vi "StateMachine.vi"() -> ()   [LabVIEW 2017]
uses:
  StateMachineController.ctl
  <vilib>/measure/mascope.llb/Amplitude and Levels 1 chan.vi
  <vilib>/Analysis/NI_AALBase.lvlib
  <vilib>/measure/NI_MAPro.lvlib
panel:
  in  "state settings":T1={"method"=enum."auto select", "histogram size"=256, "histogram method"=enum."mode", "reserved"=1.0} {"reserved" format="%0.2f"}
  out "high state level":dbl format="%.2g"
  out "amplitude":dbl format="%.2p"
  in  "Amplitude":dbl
  in  "stop":bool
  in  "Analyze Data":bool
  in  "Acquire Data":bool
  out "Waveform Graph":dbl[](graph)
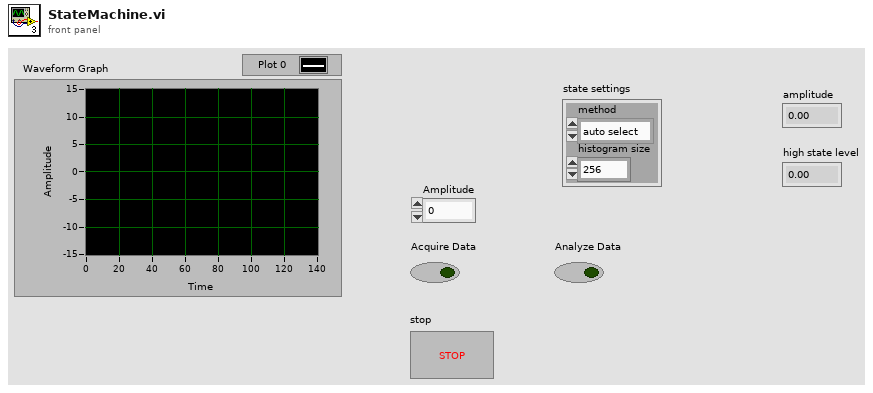
[diagram p1: front panel]
types:
  T1 = cluster{"method":enum32{"histogram", "peak", "auto select"}, "histogram size":i32, "histogram method":enum16{"mode"}, "reserved":dbl}
  T2 = typedef "StateMachineController.ctl" = enum16{"Initialize", "Stop", "Check for UI Events", "Acquire Data", "Analyze Data"}
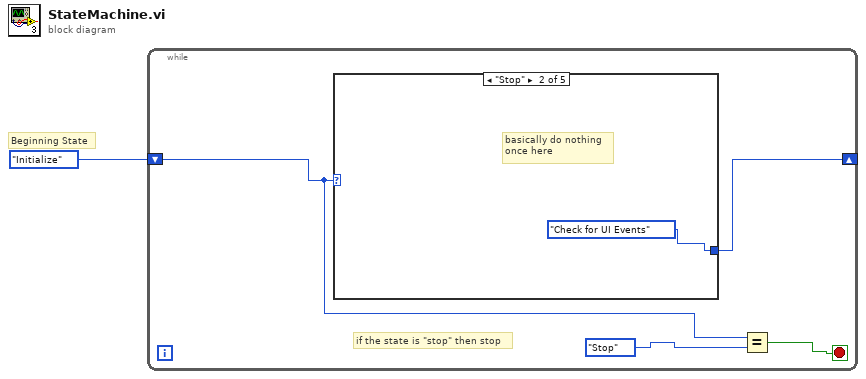
[diagram p0: block diagram]
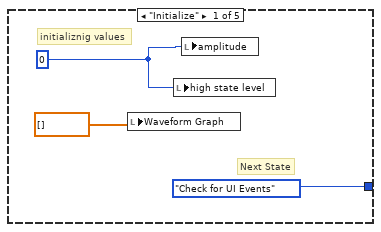
[diagram p2: hidden frame]
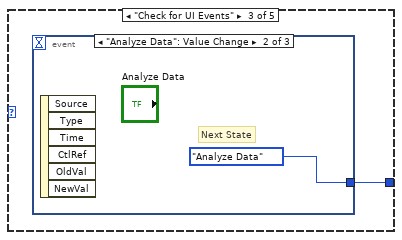
[diagram p3: hidden frame]
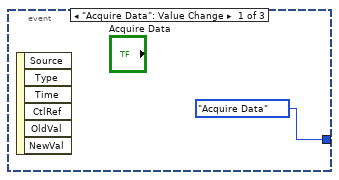
[diagram p4: hidden frame]
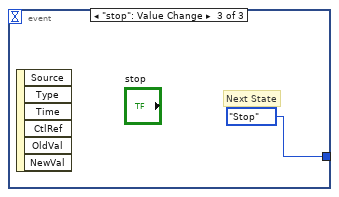
[diagram p5: hidden frame]
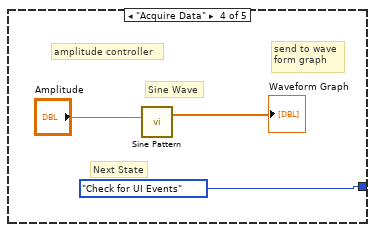
[diagram p6: hidden frame]
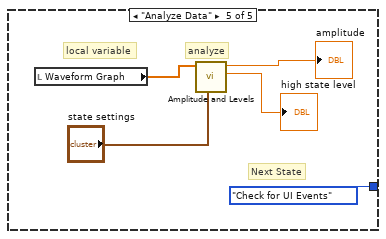
[diagram p7: hidden frame]
diagram:
  # "Beginning State"
  n1 = while {
    shift-right: [w3] -> _
    shift-left: StateMachineController."Initialize" -> [w4]
    stop <- w5 stop-if-true
    # "if the state is \"stop\" then stop"
    n2 = case shown="\"Stop\"" w4 {
      tunnel: [StateMachineController."Check for UI Events" StateMachineController."Check for UI Events" w10 StateMachineController."Check for UI Events" StateMachineController."Check for UI Events"] -> w3
      frame "Initialize" {
        w8 = 0
        # "initializnig values"
        # "Next State"
        n3 = local write "Waveform Graph"(dbl[] [] ("Waveform Graph")) -> ()
        n4 = local write "high state level"(w8) -> ()
        n5 = local write "amplitude"(w8) -> ()
      }
      frame "Stop" {
        # "basically do nothing\nonce here"
      }
      frame "Check for UI Events" {
        n6 = event shown="[1] \"Analyze Data\": Value Change" {
          selector: _ -> [_ _ _]
          dyn-events: _ -> [_ _ _]
          timeout: _ -> [_ _ _]
          tunnel: [StateMachineController."Acquire Data" StateMachineController."Analyze Data" StateMachineController."Stop"] -> w10
          event "Acquire Data": Value Change {
            n7 = event-data() -> ()  [unwired: 1 in, 6 out]
          }
          event "Analyze Data": Value Change {
            # "Next State"
            n8 = event-data() -> ()  [unwired: 1 in, 6 out]
          }
          event "stop": Value Change {
            # "Next State"
            n9 = event-data() -> ()  [unwired: 1 in, 6 out]
          }
        }
      }
      frame "Acquire Data" {
        # "send to wave\nform graph"
        # "amplitude controller"
        # "Next State"
        # "Sine Wave"
        n10 = call <vilib>:"Sine Pattern.vi"("amplitude"="Amplitude") -> ("Sinusoidal Pattern"=→"Waveform Graph":dbl[])  [unwired: 3 in, 1 out]
      }
      frame "Analyze Data" {
        # "analyze"
        # "local variable"
        # "Next State"
        n11 = local read "Waveform Graph"() -> (w21:dbl[])
        n12 = call-poly <vilib>:"Amplitude and Levels.vi"("state settings"="state settings", "signal in"=w21) -> ("high state level"=→"high state level":dbl, "amplitude"=→"amplitude":dbl)  [unwired: 6 in, 2 out]
      }
    }
    n13 = Equal?(x=w4, y=StateMachineController."Stop") -> (x = y?=w5:bool)
  }
